vi "Find Center Setup.vi"(10 "Position":dbl format="%#_13g", 11 "PUT holder in":T1) -> (3 "PUT holder out":T1)   [LabVIEW 2019, in "Pick Up Tool Fixture.lvclass"]
uses:
  Pick Up Tool Fixture.lvclass
  Find PUT holder.ctl
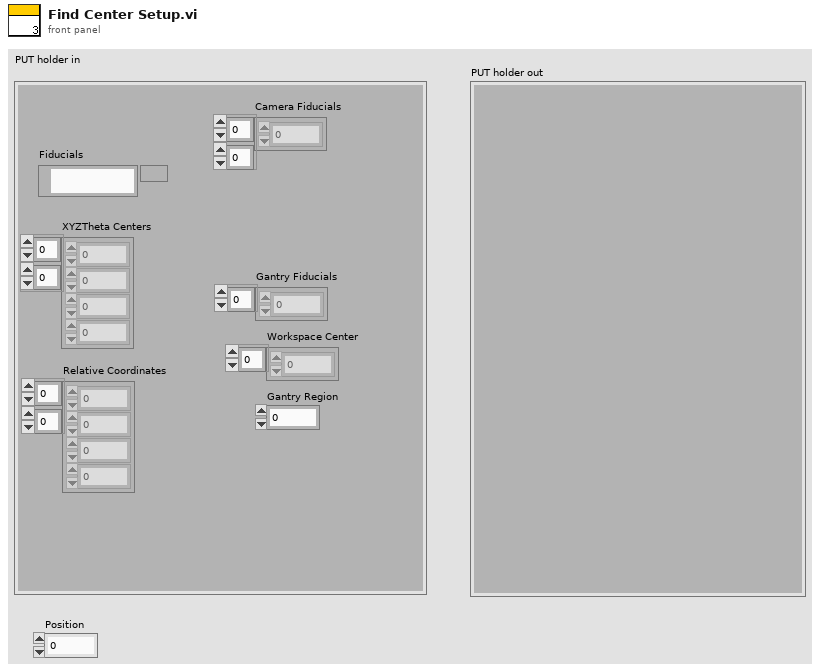
[diagram p1: front panel]
types:
  T1 = typedef "Pick Up Tool Fixture.lvclass/Find PUT holder.ctl" = cluster{"Gantry Fiducials":dbl[], "Relative Coordinates":dbl[][], "Camera Fiducials":dbl[][], "XYZTheta Centers":dbl[][], "Workspace Center":dbl[], "Gantry Region":dbl, "Fiducials":path}
  T2 = typedef "File Paths.ctl" = cluster{"Glue Pattern Folder":path, "Carrier Tray Folder":path, "Pick Up Tool Fixture Folder":path, "Components Folder":path, "Bellows Tool Offset.txt":path, "Pick Up Tool Offset.txt":path, "Dispense Tip Offset.txt":path, "Log Files":path}
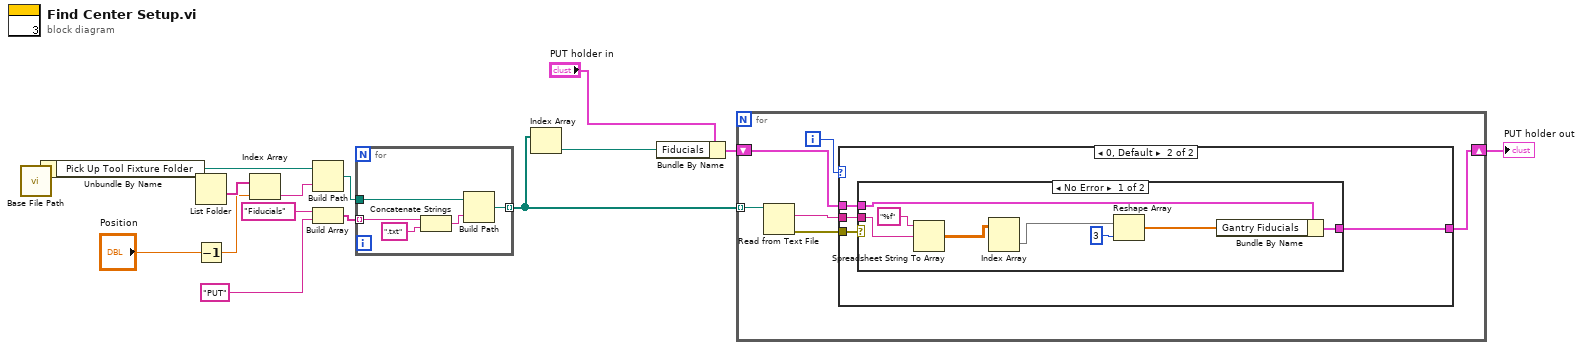
[diagram p0: block diagram]
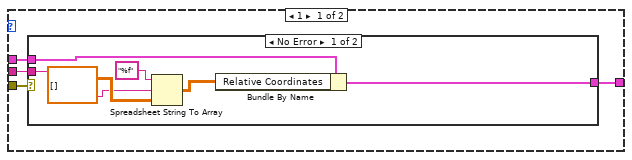
[diagram p2: hidden frame]
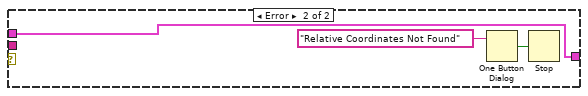
[diagram p3: hidden frame]
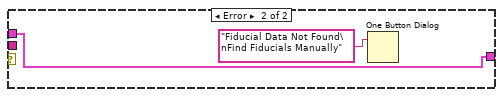
[diagram p4: hidden frame]
diagram:
  n1 = call "Base File Path.vi"() -> ("Paths Out"=w7:T2)  [unwired: 11 in]
  n2 = Unbundle By Name(w7) -> ("Pick Up Tool Fixture Folder"=w4:path)
  n3 = List Folder(path=w4) -> (folder names=w9:string[])  [unwired: 3 in, 3 out]
  n4 = Decrement(x="Position") -> (x-1=w5:dbl)
  n5 = Index Array(array=w9, index=w5) -> (element=w8:string)
  n6 = Build Path(base path=w4, name or relative path=w8) -> (appended path=w11:path)
  n7 = Build Array("Fiducials" ("format string"), "PUT" ("format string")) -> (w10:string[])
  n8 = for {
    tunnel: w10 -> [w18] mode=indexing
    tunnel: w11 -> [w20]
    tunnel: [w19] -> w3 mode=indexing
    n9 = Concatenate Strings(w18, ".txt" ("string")) -> (w16:string)
    n10 = Build Path(base path=w20, name or relative path=w16) -> (appended path=w19:path)
  }
  n11 = Index Array(array=w3) -> (element=w12:path)  [unwired: 1 in]
  n12 = Bundle By Name(cluster="PUT holder in", "Fiducials"=w12) -> (w15:T1)
  n13 = for {
    tunnel: w3 -> [w25] mode=indexing
    shift-right: [w21] -> w1
    shift-left: w15 -> [w22]
    i -> [w23]
    n14 = Read from Text File(file (use dialog)=w25) -> (text=w26:string, error out=w24:errorcluster)  [unwired: 3 in, 2 out]
    n15 = case shown="0, Default" w23 {
      tunnel: w26 -> [w29 w43]
      tunnel: w24 -> [w30 w42]
      tunnel: w22 -> [w28 w41]
      tunnel: [w27 w40] -> w21
      frame 1 {
        n16 = case shown="No Error" w30 {
          tunnel: w29 -> [w34 _]
          tunnel: [w32 w37] -> w27
          tunnel: w28 -> [w33 w37]
          frame No Error {
            n17 = Spreadsheet String To Array(format string="%f", spreadsheet string=w34, array type (2D Dbl)=dbl[][] []) -> (array=w31:dbl[][])  [unwired: 1 in]
            n18 = Bundle By Name(cluster=w33, "Relative Coordinates"=w31) -> (w32:T1)
          }
          frame Error {
            n19 = One Button Dialog(message="Relative Coordinates Not Found") -> (true=w38:bool)  [unwired: 1 in]
            n20 = Stop(stop? (T)=w38) -> ()
          }
        }
      }
      frame 0, Default {
        n21 = case shown="No Error" w42 {
          tunnel: w43 -> [w50 _]
          tunnel: w41 -> [w48 w52]
          tunnel: [w49 w52] -> w40
          frame No Error {
            n22 = Spreadsheet String To Array(format string="%f", spreadsheet string=w50) -> (array=w45:dbl[][])  [unwired: 2 in]
            n23 = Index Array(array=w45) -> (element=w44:dbl[])  [unwired: 2 in]
            n24 = Reshape Array(w44, 3 ("dimension size")) -> (w47:dbl[])
            n25 = Bundle By Name(cluster=w48, "Gantry Fiducials"=w47) -> (w49:T1)
          }
          frame Error {
            n26 = One Button Dialog(message="Fiducial Data Not Found\nFind Fiducials Manually") -> ()  [unwired: 1 in, 1 out]
          }
        }
      }
    }
  }
  "PUT holder out" <- w1
